vi "Get LV Color.vi"(8 "error in (no error)":errorcluster, 11 "RGB Color.lvclass in":refnum<class "RGB Color.lvclass">) -> (0 "error out":errorcluster, 2 "Color":u32(colorbox), 3 "RGB Color.lvclass out":refnum<class "RGB Color.lvclass">)   [LabVIEW 2018, in "RGB Color.lvclass"]
doc: "A method to get the LabVIEW color value corresponding the current color."
uses:
  RGB Color.lvclass
  RGB Color.lvclass/RGB Color.ctl
panel:
  # "expressionflow.com"
  # "Copyright (c) 2008 Tomi Maila. All rights reserved."
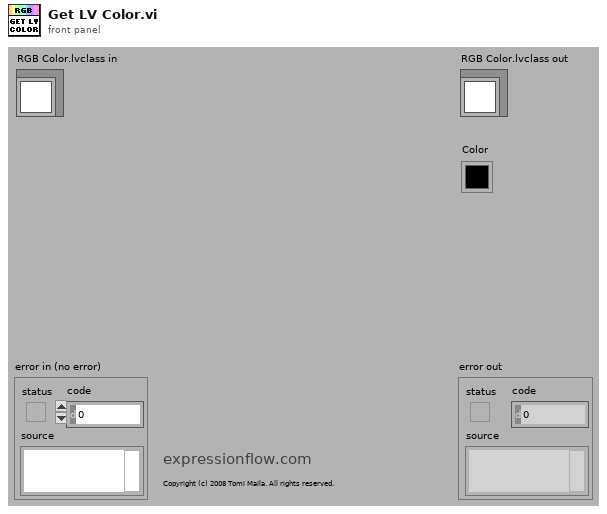
[diagram p1: front panel]
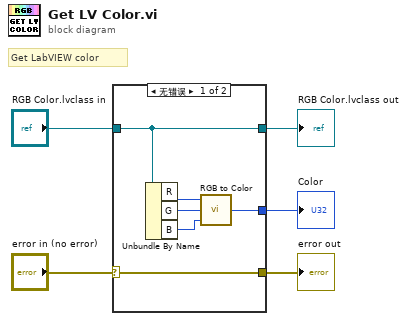
[diagram p0: block diagram]
diagram:
  # "Get LabVIEW color"
  n1 = case shown="无错误" "error in (no error)" {
    selector: "error in (no error)" -> [w11 w12]
    tunnel: [w11 w12] -> w4
    tunnel: "RGB Color.lvclass in" -> [w10 w13]
    tunnel: [w10 w13] -> w2
    tunnel: [w6 _] -> w1
    frame No Error {
      n2 = Unbundle By Name(w10) -> ("R"=w8:u8, "G"=w9:u8, "B"=w7:u8)
      n3 = call <vilib>:"RGB to Color.vi"("B"=w7, "G"=w9, "R"=w8) -> ("Color"=w6:u32)
    }
    frame Error {
    }
  }
  "error out" <- w4
  "RGB Color.lvclass out" <- w2
  "Color" <- w1
